vi "read.vi"(8 "error in (no error)":errorcluster, 11 "Lesker Pressure in":refnum<class "Lesker Pressure.lvclass">) -> (0 "error out":errorcluster, 2 "Data":dbl[](array[numeric]), 3 "Lesker Pressure out":refnum<class "Lesker Pressure.lvclass">)   [LabVIEW 2021, in "Lesker Pressure.lvclass"]
uses:
  Lesker Pressure.lvclass
  Lesker Pressure.lvclass/Lesker Pressure.ctl
  Pressure Monitor.lvclass
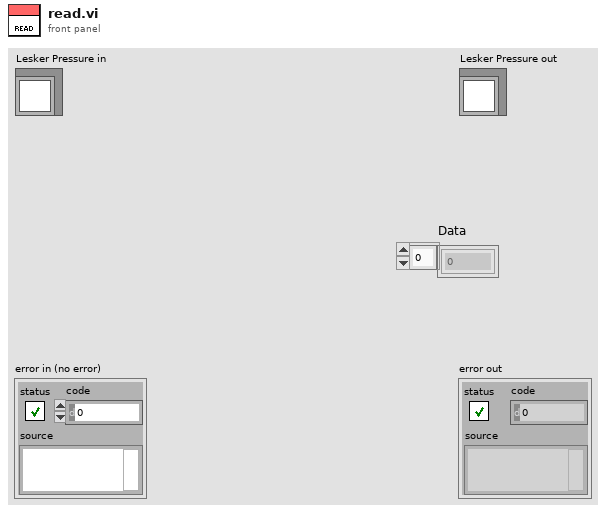
[diagram p1: front panel]
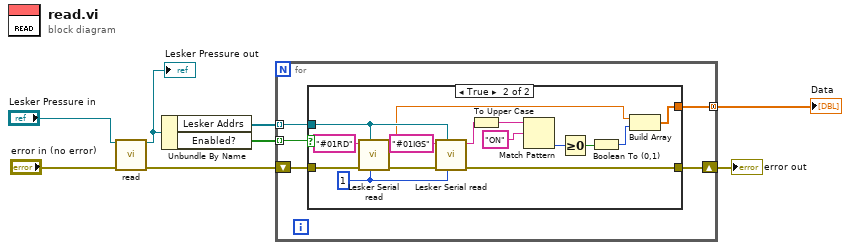
[diagram p0: block diagram]
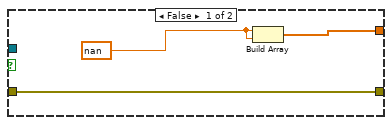
[diagram p2: hidden frame]
diagram:
  n1 = call-parent "read.vi"("error in (no error)"="error in (no error)", "Pressure Monitor in"="Lesker Pressure in") -> ("error out"=w6:errorcluster, "Pressure Monitor out"=w5:refnum<class "Lesker Pressure.lvclass">)  [unwired: 7 in, 1 out]
  "Lesker Pressure out" <- w5
  n2 = Unbundle By Name(w5) -> ("Lesker Addrs"=w3:refnum<visa-resource-name>[], "Enabled?"=w1:bool[])
  n3 = for {
    shift-right: [w12] -> w4
    shift-left: w6 -> [w13]
    tunnel: w3 -> [w11] mode=indexing
    tunnel: [w10] -> w2 mode=concatenating
    tunnel: w1 -> [w9] mode=indexing
    n4 = case shown="True" w9 {
      tunnel: w13 -> [w16 w31]
      tunnel: [w16 w28] -> w12
      tunnel: w11 -> [_ w27]
      tunnel: [w15 w18] -> w10
      frame False {
        w14 = nan ("Pressure")
        n5 = Build Array(w14, w14) -> (w15:dbl[])
      }
      frame True {
        w25 = 1 ("Number of reads")
        n6 = call "Lesker Serial read.vi"("Number of reads"=w25, "VISA resource name"=w27, "error in (no error)"=w31, "Command"="#01RD") -> ("error out"=w29:errorcluster, "Pressure"=w19:dbl)  [unwired: 5 in, 1 out]
        n7 = call "Lesker Serial read.vi"("Number of reads"=w25, "VISA resource name"=w27, "error in (no error)"=w29, "Command"="#01IGS") -> ("error out"=w28:errorcluster, "Response"=w24:string)  [unwired: 5 in, 1 out]
        n8 = To Upper Case(1:w24) -> (0:w17:string)
        n9 = Match Pattern(string=w17, regular expression="ON") -> (offset past match=w22:i32)  [unwired: 1 in, 3 out]
        n10 = Greater Or Equal To 0?(x=w22) -> (x >= 0?=w21:bool)
        n11 = Boolean To (0,1)(Boolean=w21) -> (0, 1=w20:i16)
        n12 = Build Array(w19, w20) -> (w18:dbl[])
      }
    }
  }
  "error out" <- w4
  "Data" <- w2
